vi "SanityChecker-Outputs.vi"(8 "Probe Type":u16(ring)=12 items=["5-Hole Probe"=5, "OmniProbe"=12], 10 "ReductionCode":i32[](array[numeric]), 11 "RawVmagUVWCone":dbl[][](array[numeric])) -> (0 "GoodOutputs":T1, 2 "SanitisedVmagUVWCone":dbl[][](array[numeric]), 3 "OutputErrors":T2={"PressureErrors"=[], "Plug in titles"=["Good", "AllNegative", "dPTooSmall", "P1smallest", "FailedToReduce", "ExceedMaxCone", "U.LT.0"]}, 4 "MaxCone":dbl=56.0)   [LabVIEW 2016]
uses:
  SanityCluster.ctl
  GoodArray.ctl
panel:
  out "Umin":dbl format="%#_13g"
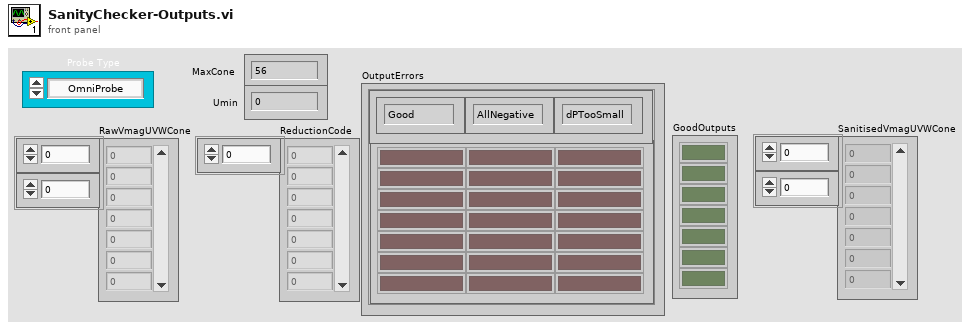
[diagram p1: front panel]
types:
  T1 = typedef "GoodArray.ctl" = bool[]
  T2 = typedef "SanityCluster.ctl" = cluster{"PressureErrors":bool[][], "Plug in titles":string[]}
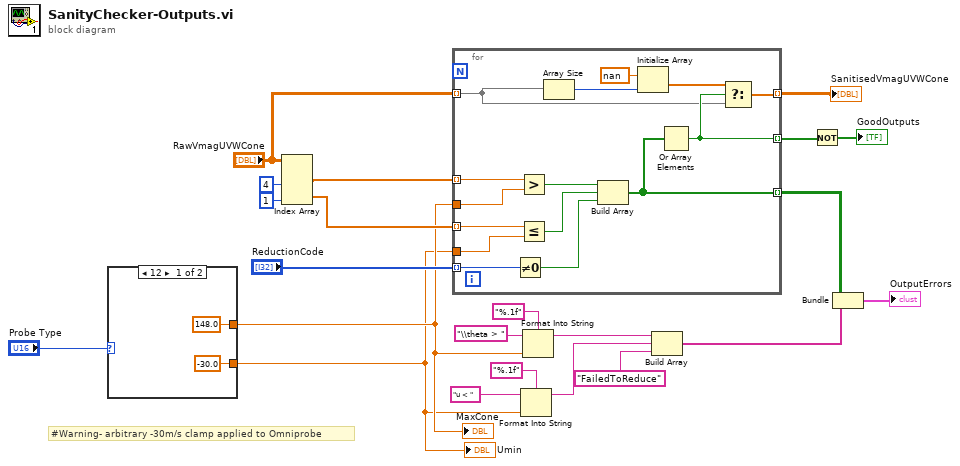
[diagram p0: block diagram]
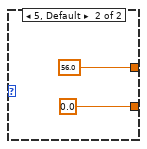
[diagram p2: hidden frame]
diagram:
  # "#Warning- arbitrary -30m/s clamp applied to Omniprobe"
  n1 = case shown="12" "Probe Type" {
    tunnel: [148.0 ("MaxCone") 56.0 ("MaxCone")] -> w2
    tunnel: [-30.0 ("Umin") 0.0 ("Umin")] -> w1
    frame 12 {
    }
    frame 5, Default {
    }
  }
  "MaxCone" <- w2
  "Umin" <- w1
  n2 = Index Array(array="RawVmagUVWCone", index (col) #1=4 ("disabled index (col)"), index (col) #2=1 ("index (col)")) -> (element #1=w12:dbl[], element #2=w11:dbl[])  [unwired: 2 in]
  n3 = for {
    tunnel: [w41] -> w9 mode=indexing
    tunnel: [w32] -> w21 mode=indexing
    tunnel: w12 -> [w38] mode=indexing
    tunnel: w11 -> [w36] mode=indexing
    tunnel: "ReductionCode" -> [w37] mode=indexing
    tunnel: w1 -> [w35]
    tunnel: w2 -> [w34]
    tunnel: [w31] -> w4 mode=indexing
    tunnel: "RawVmagUVWCone" -> [w30] mode=indexing
    n4 = Not Equal To 0?(x=w37) -> (x != 0?=w33:bool)
    n5 = Greater?(x=w38, y=w34) -> (0:w40:bool)
    n6 = Less Or Equal?(x=w36, y=w35) -> (x <= y?=w39:bool)
    n7 = Array Size(array=w30) -> (size(s)=w29:i32)
    n8 = Build Array(w40, w39, w33) -> (w41:bool[])
    n9 = Initialize Array(nan ("element"), w29) -> (w27:dbl[])
    n10 = Or Array Elements(Boolean array=w41) -> (logical OR=w32:bool)
    n11 = Select(t=w27, s=w32, f=w30) -> (s? t:f=w31:dbl[])
  }
  "SanitisedVmagUVWCone" <- w4
  n12 = Format Into String(format string="%.1f", initial string="u < ", w1) -> (resulting string=w15:string)  [unwired: 1 in, 1 out]
  n13 = Format Into String(format string="%.1f", initial string="\\theta > ", w2) -> (resulting string=w18:string)  [unwired: 1 in, 1 out]
  n14 = Build Array(w18, w15, "FailedToReduce") -> (w8:string[])
  n15 = Not(x=w21) -> (.not. x?=→"GoodOutputs":bool[])
  n16 = Bundle(w9, w8) -> (→"OutputErrors":cluster{bool[][], string[]})  [unwired: 1 in]
